vi "VIScript_UpdateTargetLangList.vi"() -> ()   [LabVIEW 2015]
panel:
  out "subarray":string[](array[string])
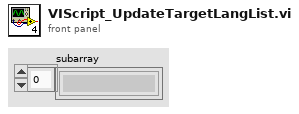
[diagram p1: front panel]
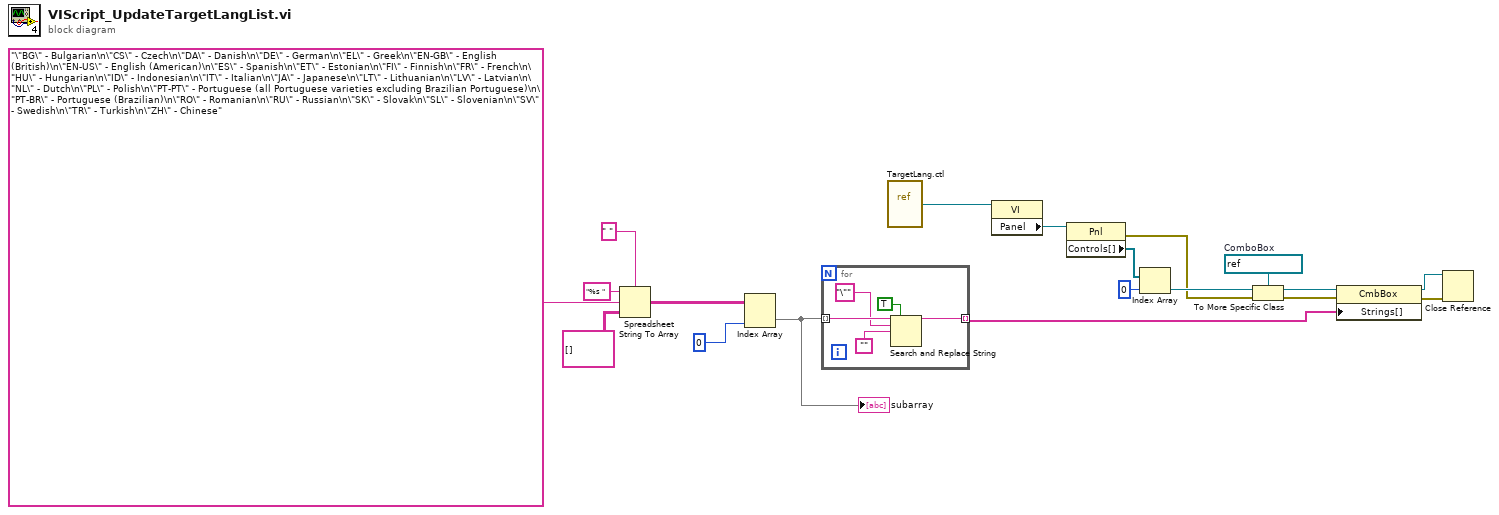
[diagram p0: block diagram]
diagram:
  w9 = refnum<vi> refnum  # ComboBox
  n1 = Spreadsheet String To Array(delimiter (Tab)=" ", format string="%s ", spreadsheet string="\"BG\" - Bulgarian\n\"CS\" - Czech\n\"DA\" - Danish\n\"DE\" - German\n\"EL\" - Greek\n\"EN-GB\" - English (British)\n\"EN-US\" - English (American)\n\"ES\" - Spanish\n\"ET\" - Estonian\n\"FI\" - Finnish\n\"FR\" - French\n\"HU\" - Hungarian\n\"ID\" - Indonesian\n\"IT\" - Italian\n\"JA\" - Japanese\n\"LT\" - Lithuanian\n\"LV\" - Latvian\n\"NL\" - Dutch\n\"PL\" - Polish\n\"PT-PT\" - Portuguese (all Portuguese varieties excluding Brazilian Portuguese)\n\"PT-BR\" - Portuguese (Brazilian)\n\"RO\" - Romanian\n\"RU\" - Russian\n\"SK\" - Slovak\n\"SL\" - Slovenian\n\"SV\" - Swedish\n\"TR\" - Turkish\n\"ZH\" - Chinese", array type (2D Dbl)=string[][] []) -> (array=w15:string[][])
  n2 = Index Array(array=w15, index (col)=0 ("disabled index (col)")) -> (element=w11:string[])  [unwired: 1 in]
  "subarray" <- w11
  n3 = for {
    tunnel: w11 -> [w24] mode=indexing
    tunnel: [w23] -> w1 mode=indexing
    n4 = Search and Replace String(replace all?=TRUE ("replace all? (F)"), input string=w24, search string="\"", replace string="") -> (result string=w23:string)  [unwired: 4 in, 3 out]
  }
  n5 = vi-ref "TargetLang.ctl"() -> (w13:refnum<vi>)
  n6 = property class="VI"(reference=w13) -> ("Panel"=w12:refnum<vi>)  [unwired: 1 in, 2 out]
  n7 = property class="Pnl"(reference=w12) -> (error out=w5:errorcluster, "Controls[]"=w10:refnum<vi>[])  [unwired: 1 in, 1 out]
  n8 = Index Array(array=w10, index=0) -> (element=w8:refnum<vi>)
  n9 = To More Specific Class(target class=w9, reference=w8, error in=w5) -> (specific class reference=w7:refnum<vi>, error out=w6:errorcluster)
  n10 = property class="CmbBox"(reference=w7, error in=w6, "Strings[]"=w1) -> (reference out=w3:refnum<vi>, error out=w2:errorcluster)
  n11 = Close Reference(reference=w3, error in (no error)=w2) -> ()  [unwired: 1 out]
